vi "数据查询_数据查询.vi"() -> ()   [LabVIEW 2016, in "数据查询.lvlib"]
uses:
  System.Windows.Forms
  <vilib>/Utility/miscctls.llb/LVPointTypeDef.ctl
  <userlib>/_OpenG.lib/array/array.llb/Sort 2D Array (String)__ogtk.vi
  <vilib>/ptbypt/NI_PtbyPt.lvlib
panel:
  in  "数据类型":string(combo)="N"
  out "columns":string[](array[string])
  out "表格":string[][](table)
  in  "剔除异常数据":bool=TRUE
  in  "WebBrowser":refnum<k24>(container)
  in  "列表框":i32(listbox)
  in  "导出":bool
  in  "测量模式":string(combo)="全部数据"
  out "选中数据表":string
  in  "查询":bool
  in  "结束日期":string="2050/01/01"
  in  "起始日期":string="2010/01/01"
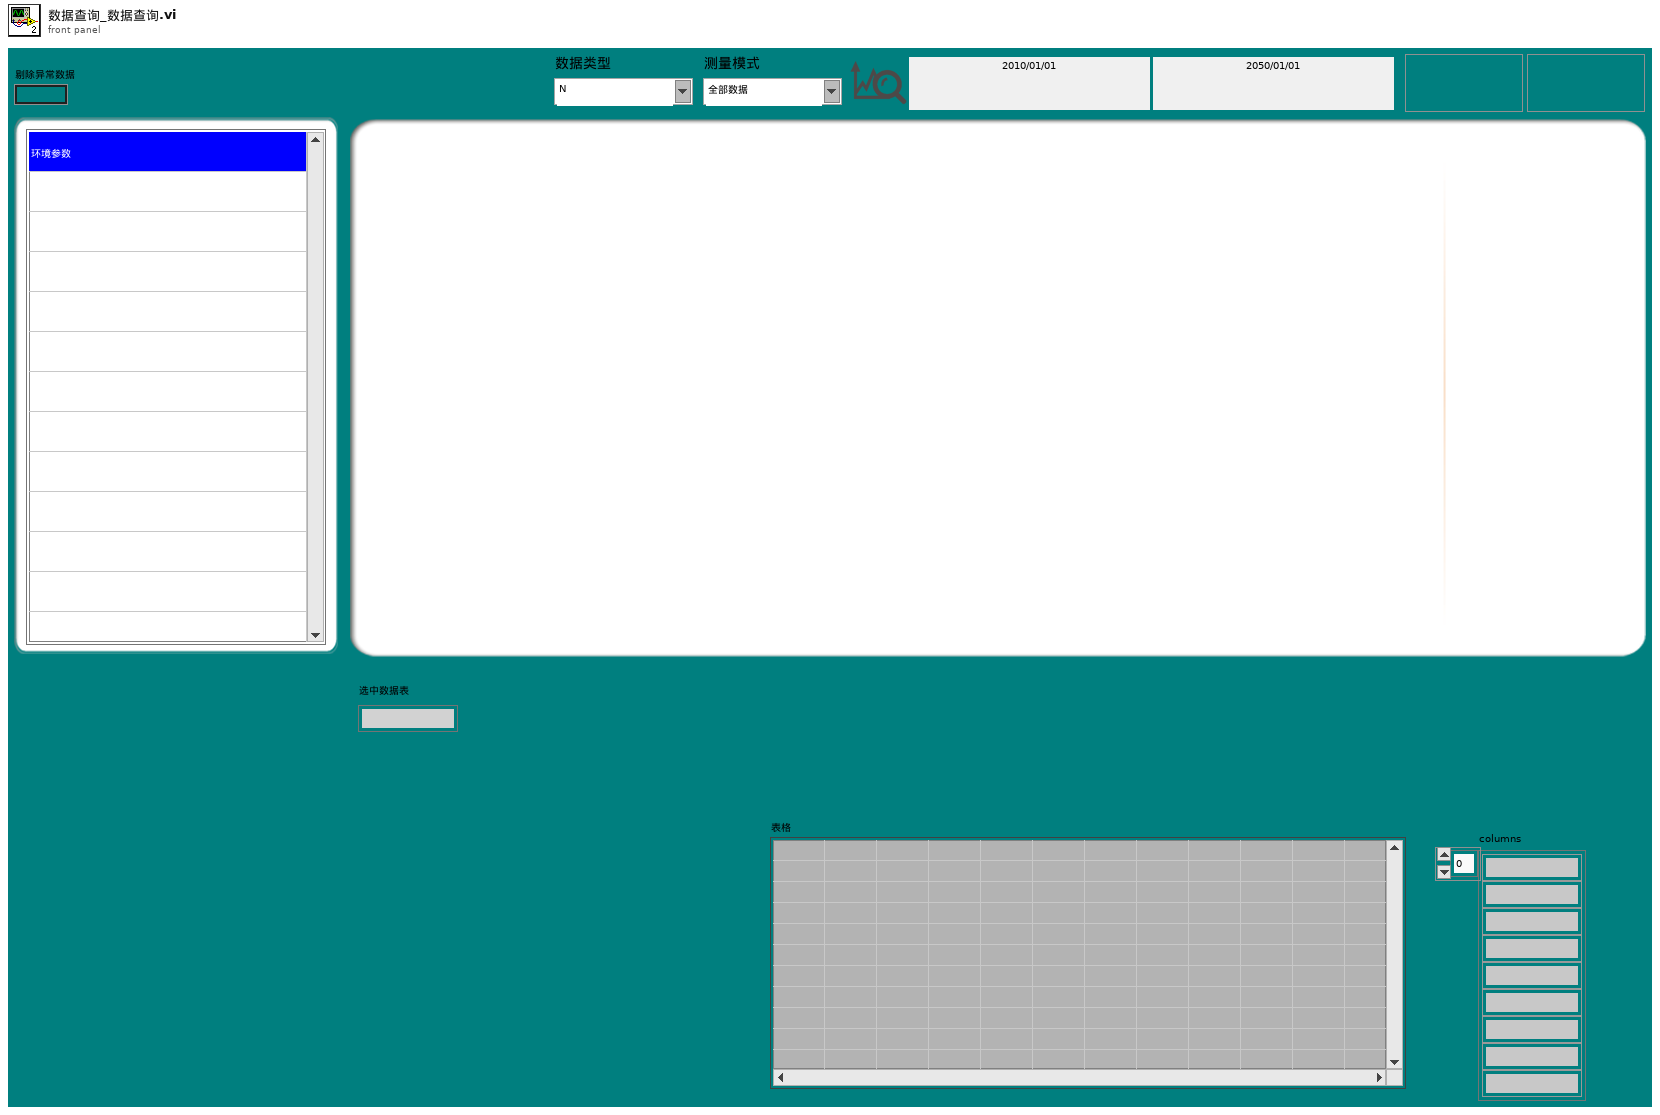
[diagram p1: front panel]
types:
  T1 = typedef "LVPointTypeDef.ctl" = cluster{"Horizontal":i16, "Vertical":i16}
  T2 = typedef "LVDateTimeRec.ctl" = cluster{"秒数的小数部分":dbl, "秒":i32, "分":i32, "时":i32, "日":i32, "月":i32, "年":i32, "天数（周）":i32, "天数（年）":i32, "DST":i32}
  T3 = typedef "数据查询.lvlib/数据查询单选控件.ctl" = enum32{"数据查询", "仪器数据", "仪器日志", "报警信息", "校准日志"}
  T4 = typedef "Rendezvous RefNum" = refnum<k1>
  T5 = enum8{"Enabled", "Disabled", "Disabled and Grayed Out"}
  T6 = typedef "数据库类型.ctl" = enum16{"Access", "SQLite"}
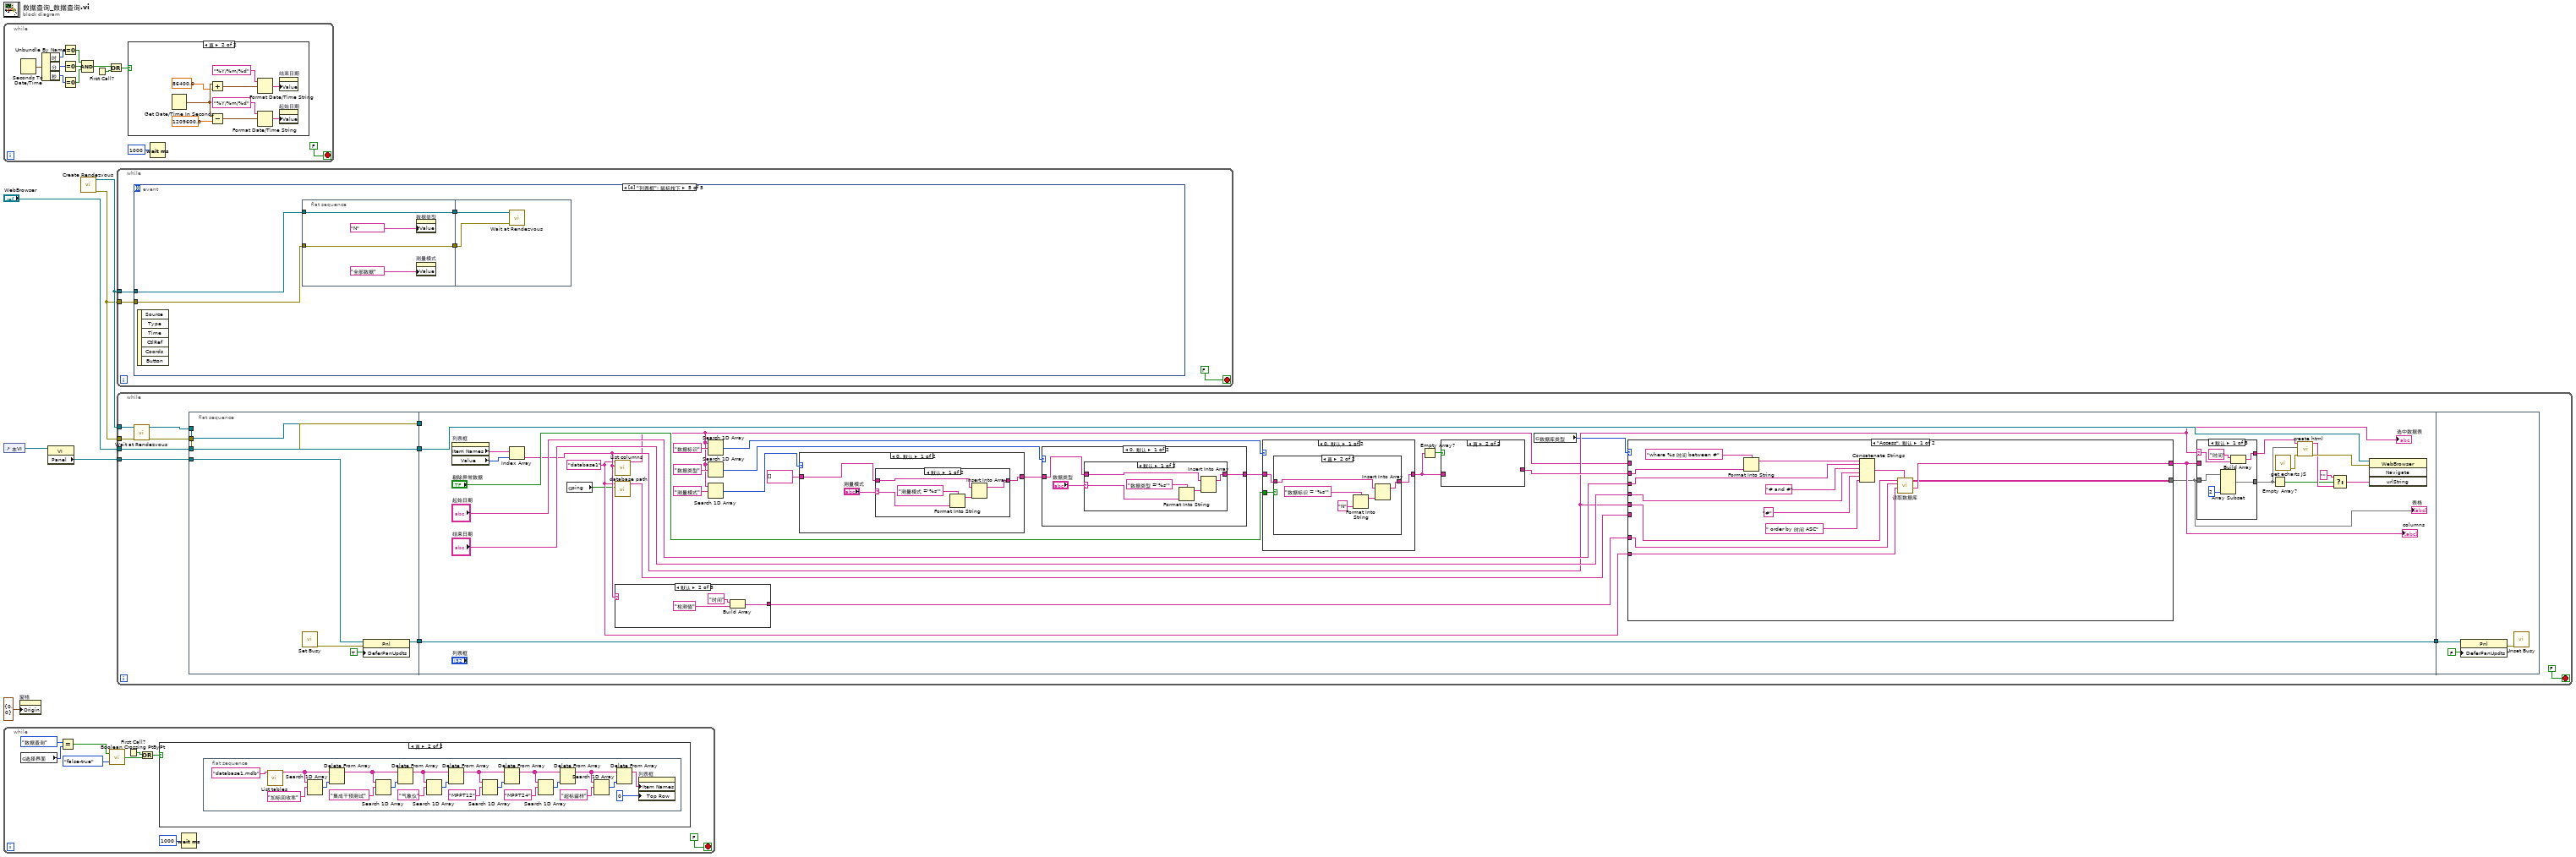
[diagram p0: block diagram]
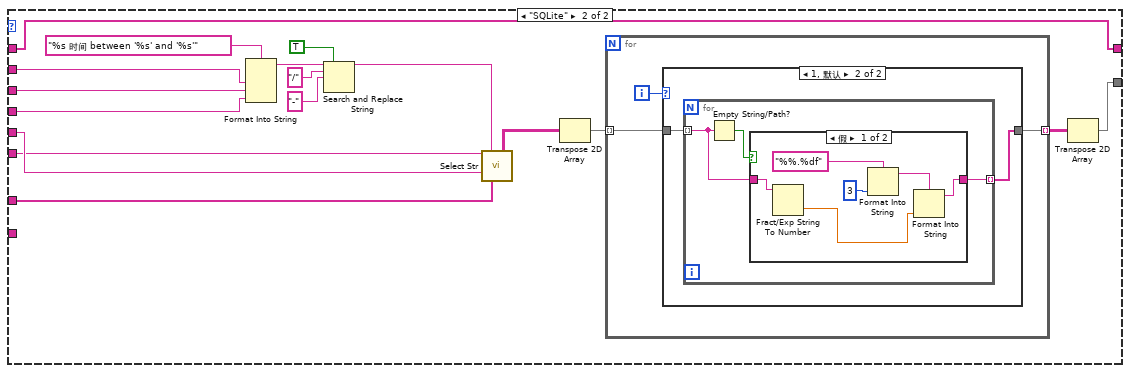
[diagram p3: hidden frame]
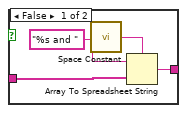
[diagram p6: hidden frame]
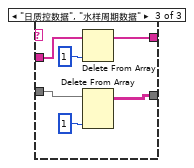
[diagram p14: hidden frame]
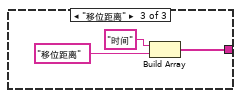
[diagram p16: hidden frame]
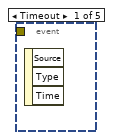
[diagram p18: hidden frame]
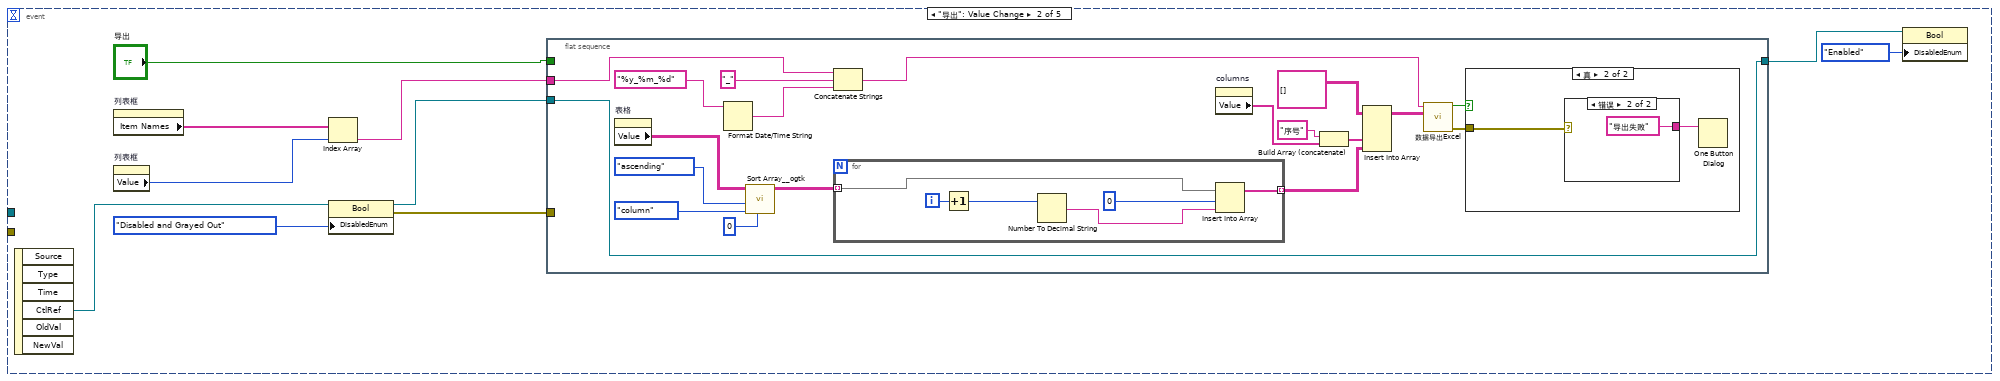
[diagram p19: hidden frame]
diagram:
  n1 = while {
    stop <- FALSE stop-if-true
    n2 = Seconds To Date/Time() -> (date time rec=w18:T2)  [unwired: 2 in]
    n3 = Unbundle By Name(w18) -> ("时"=w17:i32, "分"=w16:i32, "秒"=w15:i32)
    n4 = Equal To 0?(x=w17) -> (x = 0?=w14:bool)
    n5 = Equal To 0?(x=w16) -> (x = 0?=w13:bool)
    n6 = Equal To 0?(x=w15) -> (x = 0?=w12:bool)
    n7 = Compound Arithmetic op=AND ("复合运算")(w14, w13, w12) -> (w9:bool)
    n8 = First Call?() -> (First Call?: T/F=w7:bool)
    n9 = Or(x=w9, y=w7) -> (x .or. y?=w8:bool)
    n10 = case shown="真" w8 {
      frame False {
      }
      frame True {
        n11 = Get Date/Time In Seconds() -> (seconds since 1Jan1904=w23:timestamp)
        n12 = Add(x=w23, y=86400.0) -> (x+y=w21:timestamp)
        n13 = Subtract(x=w23, y=1209600.0) -> (x-y=w24:timestamp)
        n14 = Format Date/Time String(time format string (%c)="%Y/%m/%d" ("时间格式字符串(%c)"), seconds (now)=w21) -> (date/time string=w20:string)  [unwired: 1 in]
        n15 = Format Date/Time String(time format string (%c)="%Y/%m/%d" ("时间格式字符串(%c)"), seconds (now)=w24) -> (date/time string=w26:string)  [unwired: 1 in]
        n16 = property on="结束日期" class="Str"("Value"=w20) -> ()  [unwired: 2 in, 2 out]
        n17 = property on="起始日期" class="Str"("Value"=w26) -> ()  [unwired: 2 in, 2 out]
      }
    }
    n18 = Wait (ms)(milliseconds to wait=u32 1000 ("等待时间（毫秒）")) -> ()  [unwired: 1 out]
  }
  n19 = control-ref of="本VI"() -> (w2:refnum<vi>)
  n20 = while {
    stop <- FALSE stop-if-true
    n21 = global read "全局变量.vi" "选择界面"() -> (w34:T3)
    n22 = Equal?(x=数据查询单选控件."数据查询", y=w34) -> (x = y?=w32:bool)
    n23 = call <vilib>:"Boolean Crossing PtByPt.vi"("direction"=enum16{"either", "false-true", "true-false"}."false-true", "input"=w32) -> ("crossing"=w30:bool)  [unwired: 1 in]
    n24 = First Call?() -> (First Call?: T/F=w28:bool)
    n25 = Or(x=w28, y=w30) -> (x .or. y?=w29:bool)
    n26 = case shown="真" w29 {
      frame False {
      }
      frame True {
        n27 = flat-sequence {
          frame #0 {
            n28 = call "List tables.vi"("database"="database1.mdb") -> ("tables"=w41:string[])  [unwired: 9 in, 1 out]
            n29 = Search 1D Array(1D array=w41, element="加标回收率" ("元素")) -> (index of element=w42:i32)  [unwired: 1 in]
            n30 = Delete From Array(array=w41, index=w42) -> (array with subset deleted=w44:string[])  [unwired: 1 in, 1 out]
            n31 = Search 1D Array(1D array=w44, element="集成干预测试" ("元素")) -> (index of element=w43:i32)  [unwired: 1 in]
            n32 = Delete From Array(array=w44, index=w43) -> (array with subset deleted=w47:string[])  [unwired: 1 in, 1 out]
            n33 = Search 1D Array(1D array=w47, element="气象仪" ("元素")) -> (index of element=w45:i32)  [unwired: 1 in]
            n34 = Delete From Array(array=w47, index=w45) -> (array with subset deleted=w50:string[])  [unwired: 1 in, 1 out]
            n35 = Search 1D Array(1D array=w50, element="MPPT12" ("元素")) -> (index of element=w49:i32)  [unwired: 1 in]
            n36 = Delete From Array(array=w50, index=w49) -> (array with subset deleted=w53:string[])  [unwired: 1 in, 1 out]
            n37 = Search 1D Array(1D array=w53, element="MPPT24" ("元素")) -> (index of element=w51:i32)  [unwired: 1 in]
            n38 = Delete From Array(array=w53, index=w51) -> (array with subset deleted=w54:string[])  [unwired: 1 in, 1 out]
            n39 = Search 1D Array(1D array=w54, element="超标留样" ("元素")) -> (index of element=w56:i32)  [unwired: 1 in]
            n40 = Delete From Array(array=w54, index=w56) -> (array with subset deleted=w57:string[])  [unwired: 1 in, 1 out]
            n41 = property on="列表框" class="LstBox (严格)"("Item Names"=w57, "Top Row"=0 ("顶行")) -> ()  [unwired: 2 in, 2 out]
          }
        }
      }
    }
    n42 = Wait (ms)(milliseconds to wait=u32 1000 ("等待时间（毫秒）")) -> ()  [unwired: 1 out]
  }
  n43 = property on="窗格" class="Pane"("Origin"=T1 {"Horizontal"=0, "Vertical"=0} ("原点")) -> ()  [unwired: 2 in, 2 out]
  n44 = property class="VI"(reference=w2) -> ("Panel"=w1:refnum<vi>)  [unwired: 1 in, 2 out]
  n45 = call <vilib>:"Create Rendezvous.vi"() -> ("error out"=w3:errorcluster, "rendezvous"=w4:T4)  [unwired: 5 in, 1 out]
  n46 = while {
    tunnel: w4 -> [w59]
    tunnel: w3 -> [w58]
    stop <- FALSE stop-if-true
    n47 = event shown="[4] \"列表框\": 鼠标按下" {
      selector: _ -> [_ _ _ _ _]
      dyn-events: _ -> [_ _ _ _ _]
      timeout: _ -> [_ _ _ _ _]
      tunnel: w59 -> [_ _ _ w105 w108]
      tunnel: w58 -> [_ _ _ w104 w106]
      event Timeout {
        n48 = event-data() -> ()  [unwired: 1 in, 3 out]
      }
      event "导出": Value Change {
        n49 = event-data() -> ("CtlRef"=w70:refnum<vi>)  [unwired: 1 in, 5 out]
        n50 = property on="列表框" class="LstBox (严格)"() -> ("Item Names"=w63:string[])  [unwired: 2 in, 2 out]
        n51 = property on="列表框" class="LstBox (严格)"() -> ("Value"=w62:i32)  [unwired: 2 in, 2 out]
        n52 = Index Array(array=w63, index=w62) -> (element=w61:string)
        n53 = property class="Bool"(reference=w70, "DisabledEnum"=T5."Disabled and Grayed Out" ("禁用")) -> (reference out=w67:refnum<vi>, error out=w68:errorcluster)  [unwired: 1 in]
        n54 = flat-sequence {
          tunnel: w68 -> [_]
          tunnel: [w86] -> w66
          tunnel: w67 -> [w86]
          tunnel: "导出" -> [_]
          tunnel: w61 -> [w76]
          frame #0 {
            n55 = property on="表格" class="Tbl (严格)"() -> ("Value"=w72:string[][])  [unwired: 2 in, 2 out]
            n56 = Format Date/Time String(time format string (%c)="%y_%m_%d" ("时间格式字符串(%c)")) -> (date/time string=w83:string)  [unwired: 2 in]
            n57 = call-poly <userlib>:"Sort Array__ogtk.vi"("Column/Row to Sort By"=u32 0, "Sort By in"=enum16{"row", "column"}."column", "Order"=enum16{"ascending", "descending"}."ascending", "Array in"=w72) -> ("Sorted Array out"=w80:string[][])  [unwired: 4 in, 3 out]
            n58 = Concatenate Strings(w76, "_" ("字符串"), w83) -> (w81:string)
            n59 = for {
              tunnel: w80 -> [w98] mode=indexing
              tunnel: [w97] -> w73 mode=indexing
              i -> [w99]
              n60 = Increment(x=w99) -> (x+1=w95:i32)
              n61 = Number To Decimal String(number=w95) -> (decimal integer string=w94:string)  [unwired: 1 in]
              n62 = Insert Into Array(array=w98, index=0 ("索引"), new element=w94) -> (w97:string[])
            }
            n63 = property on="columns" class="Arr (严格)"() -> ("Value"=w71:string[])  [unwired: 2 in, 2 out]
            n64 = Build Array (concatenate)("序号" ("新元素/子数组"), w71) -> (w74:string[])
            n65 = Insert Into Array(array=string[][] [], new element #1=w74, new element #2=w73) -> (w79:string[][])  [unwired: 2 in]
            n66 = call "数据导出Excel.vi"("text data"=w79, "default name"=w81) -> ("error out"=w78:errorcluster, "布尔"=w77:bool)  [unwired: 8 in]
            n67 = case shown="真" w77 {
              tunnel: w78 -> [_ w91]
              frame False {
              }
              frame True {
                n68 = case shown="错误" w91 {
                  tunnel: ["导出成功" ("消息") "导出失败" ("消息")] -> w90
                  frame No Error {
                  }
                  frame Error {
                  }
                }
                n69 = One Button Dialog(message=w90) -> ()  [unwired: 1 in, 1 out]
              }
            }
          }
        }
        n70 = property class="Bool"(reference=w66, "DisabledEnum"=T5."Enabled" ("禁用")) -> ()  [unwired: 1 in, 2 out]
      }
      event "起始日期", "结束日期": Mouse Down {
        n71 = event-data() -> ("CtlRef"=w103:refnum<vi>)  [unwired: 1 in, 7 out]
        n72 = property class="Str"(reference=w103) -> (reference out=w101:refnum<vi>, "Value"=w102:string)  [unwired: 1 in, 1 out]
        n73 = call "日期键盘.vi"("原值"=w102) -> ("x+y"=w100:string)  [unwired: 10 in]
        n74 = property class="Str"(reference=w101, "Val(Sgnl)"=w100) -> ()  [unwired: 1 in, 2 out]
      }
      event "查询", "起始日期", "结束日期", "测量模式", "剔除异常数据", "数据类型": Value Change {
        n75 = event-data() -> ()  [unwired: 1 in, 6 out]
        n76 = call <vilib>:"Wait at Rendezvous.vi"("error in (no error)"=w104, "rendezvous"=w105) -> ()  [unwired: 3 in, 3 out]
      }
      event "列表框": Mouse Down {
        n77 = event-data() -> ()  [unwired: 1 in, 6 out]
        n78 = flat-sequence {
          tunnel: [w111] -> w109
          tunnel: w108 -> [w111]
          tunnel: [w110] -> w107
          tunnel: w106 -> [w110]
          tunnel: w109 -> [w115]
          tunnel: w107 -> [w114]
          frame #0 {
            n79 = property on="数据类型" class="CmbBox"("Value"="N" ("数据类型")) -> ()  [unwired: 2 in, 2 out]
            n80 = property on="测量模式" class="CmbBox"("Value"="全部数据" ("测量模式")) -> ()  [unwired: 2 in, 2 out]
          }
          frame #1 {
            n81 = call <vilib>:"Wait at Rendezvous.vi"("error in (no error)"=w114, "rendezvous"=w115) -> ()  [unwired: 3 in, 3 out]
          }
        }
      }
    }
  }
  n82 = while {
    tunnel: "WebBrowser" -> [w126]
    tunnel: w4 -> [w125]
    tunnel: w3 -> [w124]
    tunnel: w1 -> [w118]
    stop <- FALSE stop-if-true
    n83 = call <vilib>:"Wait at Rendezvous.vi"("error in (no error)"=w124, "rendezvous"=w125) -> ("error out"=w123:errorcluster, "rendezvous out"=w122:T4)  [unwired: 3 in, 1 out]
    n84 = flat-sequence {
      tunnel: w122 -> [w132]
      tunnel: w123 -> [w133]
      tunnel: w126 -> [w134]
      tunnel: [w134] -> w121
      tunnel: [w133] -> w120
      tunnel: [w132] -> w119
      tunnel: w118 -> [w131]
      tunnel: [w129] -> w117
      tunnel: w121 -> [w168]
      tunnel: w120 -> [_]
      tunnel: w119 -> [_]
      tunnel: w117 -> [w135]
      tunnel: [w135] -> w116
      tunnel: w116 -> [w274]
      frame #0 {
        n85 = call <vilib>:"Set Busy.vi"() -> ("error out"=w128:errorcluster)  [unwired: 10 in, 1 out]
        n86 = property class="Pnl"(reference=w131, error in=w128, "DeferPanUpdts"=TRUE ("延迟前面板更新")) -> (reference out=w129:refnum<vi>)  [unwired: 1 out]
      }
      frame #1 {
        w138 = "database1" ("database")
        n87 = property on="列表框" class="LstBox (严格)"() -> ("Item Names"=w160:string[], "Value"=w159:i32)  [unwired: 2 in, 2 out]
        n88 = Index Array(array=w160, index=w159) -> (element=w151:string)
        "选中数据表" <- w151
        n89 = global read "全局变量.vi" "ping"() -> (w137:bool)
        n90 = call "List columns.vi"("table"=w151, "database"=w138) -> ("columns"=w140:string[])  [unwired: 8 in, 1 out]
        n91 = call "database path.vi"("ping"=w137, "database"=w138) -> ("Path out"=w139:string)  [unwired: 8 in, 1 out]
        n92 = case shown="默认" w151 {
          tunnel: [_ w266 w269] -> w162
          frame "多参数", "环境参数", "日质控数据", "水样周期数据" {
          }
          frame Default {
            n93 = Build Array("时间", "检测值") -> (w266:string[])
          }
          frame "移位距离" {
            n94 = Build Array("时间", "移位距离") -> (w269:string[])
          }
        }
        n95 = Search 1D Array(1D array=w140, element="数据标识" ("元素")) -> (index of element=w143:i32)  [unwired: 1 in]
        n96 = Search 1D Array(1D array=w140, element="数据类型" ("元素")) -> (index of element=w144:i32)  [unwired: 1 in]
        n97 = Search 1D Array(1D array=w140, element="测量模式" ("元素")) -> (index of element=w146:i32)  [unwired: 1 in]
        n98 = case shown="0, 默认" w146 {
          tunnel: string[] [] -> [w244 w251]
          tunnel: [w242 w251] -> w145
          frame 0, Default {
            n99 = case shown="默认" "测量模式" {
              selector: "测量模式" -> [w245 _]
              tunnel: w244 -> [w248 w250]
              tunnel: [w246 w250] -> w242
              frame Default {
                n100 = Format Into String(format string="测量模式 ='%s'" ("condition"), w245) -> (resulting string=w247:string)  [unwired: 2 in, 1 out]
                n101 = Insert Into Array(array=w248, new element=w247) -> (w246:string[])  [unwired: 1 in]
              }
              frame "全部数据" {
              }
            }
          }
          frame -1 {
          }
        }
        n102 = case shown="0, 默认" w144 {
          tunnel: [w233 w241] -> w147
          tunnel: w145 -> [w232 w241]
          frame 0, Default {
            n103 = case shown="默认" "数据类型" {
              selector: "数据类型" -> [w235 _]
              tunnel: w232 -> [w238 w240]
              tunnel: [w236 w240] -> w233
              frame Default {
                n104 = Format Into String(format string="数据类型 ='%s'" ("condition"), w235) -> (resulting string=w237:string)  [unwired: 2 in, 1 out]
                n105 = Insert Into Array(array=w238, new element=w237) -> (w236:string[])  [unwired: 1 in]
              }
              frame "全部数据" {
              }
            }
          }
          frame -1 {
          }
        }
        n106 = case shown="0, 默认" w143 {
          tunnel: "剔除异常数据" -> [w224 _]
          tunnel: [w223 w231] -> w142
          tunnel: w147 -> [w222 w231]
          frame 0, Default {
            n107 = case shown="真" w224 {
              tunnel: w222 -> [w225 w230]
              tunnel: [w225 w229] -> w223
              frame False {
              }
              frame True {
                n108 = Format Into String(format string="数据标识 = '%s'" ("condition"), "N" ("String")) -> (resulting string=w226:string)  [unwired: 2 in, 1 out]
                n109 = Insert Into Array(array=w230, new element=w226) -> (w229:string[])  [unwired: 1 in]
              }
            }
          }
          frame -1 {
          }
        }
        n110 = Empty Array?(array=w142) -> (empty?=w141:bool)
        n111 = case shown="真" w141 {
          tunnel: [w221 _] -> w152
          tunnel: w142 -> [w218 _]
          frame False {
            n112 = call <vilib>:"Space Constant.vi"() -> ("String"=w220:string)
            n113 = Array To Spreadsheet String(delimiter (Tab)=w220, array=w218, 3:"%s and " ("格式字符串")) -> (spreadsheet string=w221:string)
          }
          frame True {
          }
        }
        n114 = global read "外部调用接口全局变量.vi" "数据库类型"() -> (w136:T6)
        n115 = case shown="\"Access\", 默认" w136 {
          tunnel: "结束日期" -> [w180 w192]
          tunnel: "起始日期" -> [w179 w193]
          tunnel: [w178 w190] -> w165
          tunnel: [w177 w191] -> w163
          tunnel: w162 -> [w176 w186]
          tunnel: w152 -> [w175 w194]
          tunnel: w151 -> [w172 w187]
          tunnel: w140 -> [_ w190]
          tunnel: w139 -> [_ w185]
          tunnel: w138 -> [w171 _]
          frame "Access", Default {
            n116 = Format Into String(format string="where %s 时间 between #" ("condition"), w175) -> (resulting string=w173:string)  [unwired: 2 in, 1 out]
            n117 = Concatenate Strings(w173, w179, "# and #" ("condition"), w180, "#" ("condition"), " order by 时间 ASC" ("字符串")) -> (w184:string)
            n118 = call "读取数据库.vi"("condition"=w184, "database"=w171, "显示项"=w176, "组合框"=w172) -> ("columns"=w178:string[], "表格"=w177:string[][])  [unwired: 4 in, 2 out]
          }
          frame "SQLite" {
            n119 = Format Into String(format string="%s 时间 between '%s' and '%s'" ("格式字符串"), w194, w193, w192) -> (resulting string=w197:string)  [unwired: 2 in, 1 out]
            n120 = Search and Replace String(replace all?=TRUE ("替换全部？(F)"), input string=w197, search string="/" ("搜索字符串"), replace string="-" ("替换字符串(\"\")")) -> (result string=w189:string)  [unwired: 4 in, 3 out]
            n121 = call "Select Str.vi"("DB Path"=w185, "Where Clause"=w189, "Tables Name"=w187, "Columns"=w186) -> ("Results"=w188:string[][])  [unwired: 8 in, 3 out]
            n122 = Transpose 2D Array(2D array=w188) -> (transposed array=w196:string[][])
            n123 = for {
              tunnel: w196 -> [w204] mode=indexing
              tunnel: [w203] -> w195 mode=indexing
              i -> [w202]
              n124 = case shown="1, 默认" w202 {
                tunnel: w204 -> [w205 w207]
                tunnel: [w205 w206] -> w203
                frame 0 {
                }
                frame 1, Default {
                  n125 = for {
                    tunnel: w207 -> [w209] mode=indexing
                    tunnel: [w210] -> w206 mode=indexing
                    n126 = Empty String/Path?(string/path=w209) -> (empty?=w208:bool)
                    n127 = case shown="假" w208 {
                      tunnel: [w214 w217] -> w210
                      tunnel: w209 -> [w211 w217]
                      frame False {
                        n128 = Fract/Exp String To Number(string=w211) -> (number=w213:dbl)  [unwired: 3 in, 1 out]
                        n129 = Format Into String(format string="%%.%df" ("格式字符串"), 3 ("输入 1")) -> (resulting string=w216:string)  [unwired: 2 in, 1 out]
                        n130 = Format Into String(format string=w216, w213) -> (resulting string=w214:string)  [unwired: 2 in, 1 out]
                      }
                      frame True {
                      }
                    }
                  }
                }
              }
            }
            n131 = Transpose 2D Array(2D array=w195) -> (transposed array=w191:string[][])
          }
        }
        "表格" <- w163
        "columns" <- w165
        n132 = case shown="默认" w151 {
          selector: w151 -> [w254 _ _]
          tunnel: w165 -> [_ w259 w265]
          tunnel: [w253 w259 w264] -> w164
          tunnel: w163 -> [w257 w258 w262]
          tunnel: [w256 w258 w261] -> w155
          frame Default {
            n133 = Array Subset(array=w257, length (col)=2 ("长度")) -> (w256:string[][])  [unwired: 3 in]
            n134 = Build Array("时间", w254) -> (w253:string[])
          }
          frame "多参数", "环境参数" {
          }
          frame "日质控数据", "水样周期数据" {
            n135 = Delete From Array(array=w265, index=1 ("索引")) -> (array with subset deleted=w264:string[])  [unwired: 1 in, 1 out]
            n136 = Delete From Array(array=w262, index (col)=1 ("禁用的索引 (列)")) -> (array with subset deleted=w261:string[][])  [unwired: 2 in, 1 out]
          }
        }
        n137 = Empty Array?(array=w155) -> (empty?=w154:bool)
        n138 = call "get echarts JS.vi"() -> ("error out"=w167:errorcluster)  [unwired: 11 in]
        n139 = call "create html.vi"("error in (no error)"=w167, "data"=w155, "columns"=w164) -> ("error out"=w166:errorcluster, "url"=w158:string)  [unwired: 7 in]
        n140 = Select(t="", s=w154, f=w158) -> (s? t:f=w157:string)
        n141 = invoke class="WebBrowser" method="Navigate"(reference=w168, error in=w166, "urlString"=w157) -> ()  [unwired: 1 in, 4 out]
      }
      frame #2 {
        n142 = property class="Pnl"(reference=w274, "DeferPanUpdts"=FALSE ("延迟前面板更新")) -> (error out=w272:errorcluster)  [unwired: 1 in, 1 out]
        n143 = call <vilib>:"Unset Busy.vi"("error in (no error)"=w272) -> ()  [unwired: 10 in, 1 out]
      }
    }
  }
